vi "Finalize.vi"(8 "error in":errorcluster, 11 "Plugin in":refnum<class "PXIe4113 DUT Power Control Replacement.lvclass">) -> (0 "error out":errorcluster, 3 "Plugin out":refnum<class "PXIe4113 DUT Power Control Replacement.lvclass">)   [LabVIEW 2026, in "PXIe4113 DUT Power Control Replacement.lvlib" / "PXIe4113 DUT Power Control Replacement.lvclass"]
uses:
  PXIe4113 DUT Power Control Replacement.lvclass
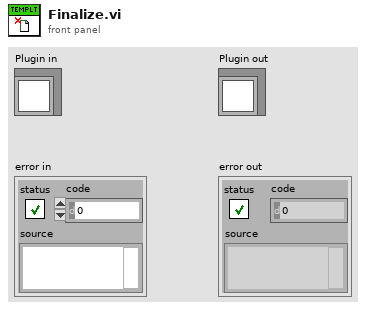
[diagram p1: front panel]
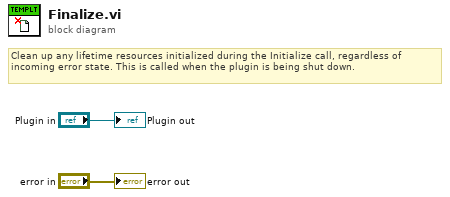
[diagram p0: block diagram]
diagram:
  # "Clean up any lifetime resources initialized during the Initialize call, regardless of incoming error state. This is called when the plugin is being shut down."
  "error out" <- "error in"
  "Plugin out" <- "Plugin in"
